vi "LabJackT4_Main.vi"() -> ()   [LabVIEW 2019]
uses:
  sub/enum_dev_id.ctl
  <vilib>/Analysis/baseanly.llb/Mean (DBL).vi
  <vilib>/Analysis/NI_AALBase.lvlib
panel:
  in  "logging_on":bool=TRUE
  out "status":bool
  out "TC_avg_degF":dbl format="%.1f"
  out "TC_avg_degC":dbl format="%.1f"
  out "array_ref_temp":dbl[](array[numeric]) caption="CJC" format="%_4g"
  out "Pressure":dbl
  in  "Tab Control":T1(tab)
  out "chart_pres":waveform(dbl)[](graph)=[{"t0"=timestamp(3772890114.31303 s since 1904-01-01), "dt"=1.0, "Y"=[0.8687935985565186]}, {"t0"=timestamp(3772890114.31303 s since 1904-01-01), "dt"=1.0, "Y"=[86.87935985565186]}, {"t0"=timestamp(3772890114.31303 s since 1904-01-01), "dt"=1.0, "Y"=[30.48853325313992]}, {"t0"=timestamp(3772890114.31303 s since 1904-01-01), "dt"=1.0, "Y"=[303.6385332531399]}]
  in  "SPTD25":string="AIN0"
  out "Chart degF":waveform(dbl)[](graph)
  out "Chart degC":waveform(dbl)[](graph)
  in  "LM34CAZ":string="AIN2"
  out "chart_ref_temp":waveform(dbl)[](graph)=[{"t0"=timestamp(3772890114.31303 s since 1904-01-01), "dt"=1.0, "Y"=[0.8687935985565186]}, {"t0"=timestamp(3772890114.31303 s since 1904-01-01), "dt"=1.0, "Y"=[86.87935985565186]}, {"t0"=timestamp(3772890114.31303 s since 1904-01-01), "dt"=1.0, "Y"=[30.48853325313992]}, {"t0"=timestamp(3772890114.31303 s since 1904-01-01), "dt"=1.0, "Y"=[303.6385332531399]}]
  out "chart_raw_v":waveform(dbl)[](graph)
  out "avg_data":dbl[](array[numeric])
  out "array_TC_degF":dbl[](array[numeric]) caption="TC degF" format="%_4g"
  out "array_TC_mV":dbl[](array[numeric]) caption="TC mV" format="%_4f"
  in  "amp_gain":dbl[](array[numeric])=[260.2, 260.0, 259.9, 259.8] format="%_4f"
  in  "amp_offset":dbl[](array[numeric])=[1.2648, 1.2687, 1.2357, 1.2546] format="%_5g"
  out "array_TC_degC":dbl[](array[numeric]) caption="TC degC" format="%_4g"
  in  "clear_chart":bool caption="Clear charts to start"
  in  "dev_id":T2=enum."192.168.24.185"
  out "SN":i32
  in  "conn_type":T3(ring)=enum."LJM_ctETHERNET"
  out "Last Meas. Time":timestamp format="%<%Y-%m-%d %H:%M:%S>T"
  in  "Read Rate (Hz)":dbl=0.1 format="%#_15g"
  out "iter":i32 caption="Meas. count"
  in  "Scan Rate (Hz)":dbl=5000.0 format="%#.3f"
  in  "stop":bool
  out "Error Message":string
  # "Pressure & Temperature of Outside gHe Tank"
  # "LabJack T4"
  # "psi"
  # "CH4"
  # "V"
  # "Bottom"
  # "degF"
  # "CH5"
  # "Right"
  # "CH6"
  # "Top"
  # "degC"
  # "CH7"
  # "K"
  # "Left"
  # "Average"
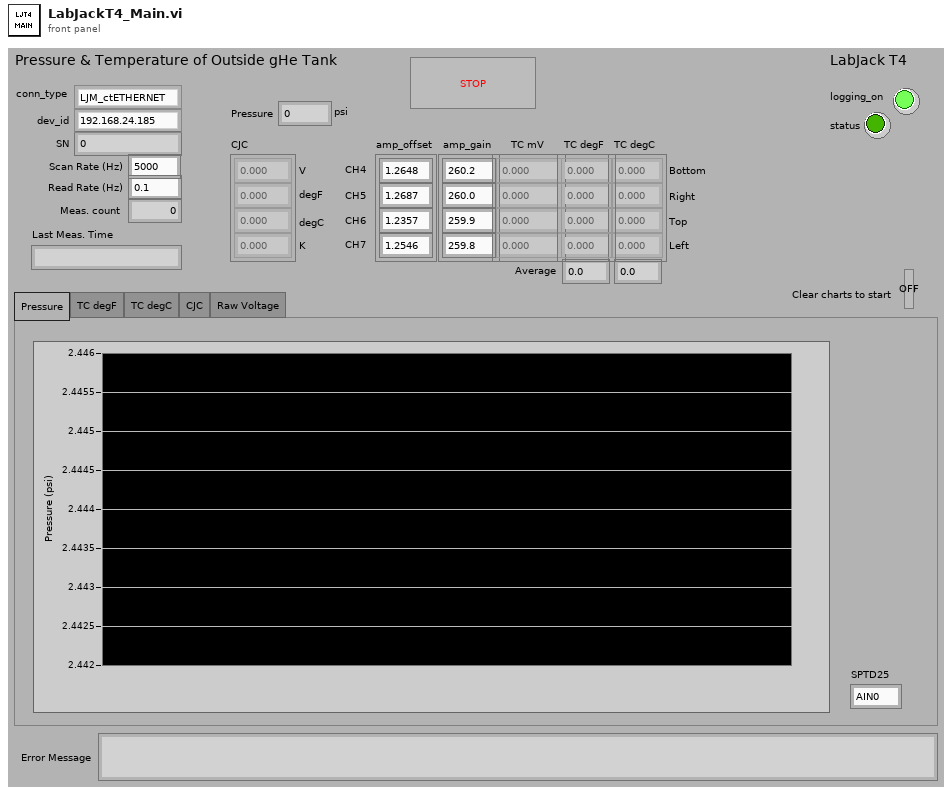
[diagram p1: front panel]
types:
  T1 = enum32{"Pressure", "TC degF", "TC degC", "CJC", "Raw Voltage"}
  T2 = typedef "enum_dev_id.ctl" = enum16{"LJM_idANY", "192.168.24.185", "10.0.0.176", "440017305"}
  T3 = enum16{"LJM_ctANY", "LJM_ctUSB", "LJM_ctETHERNET"}
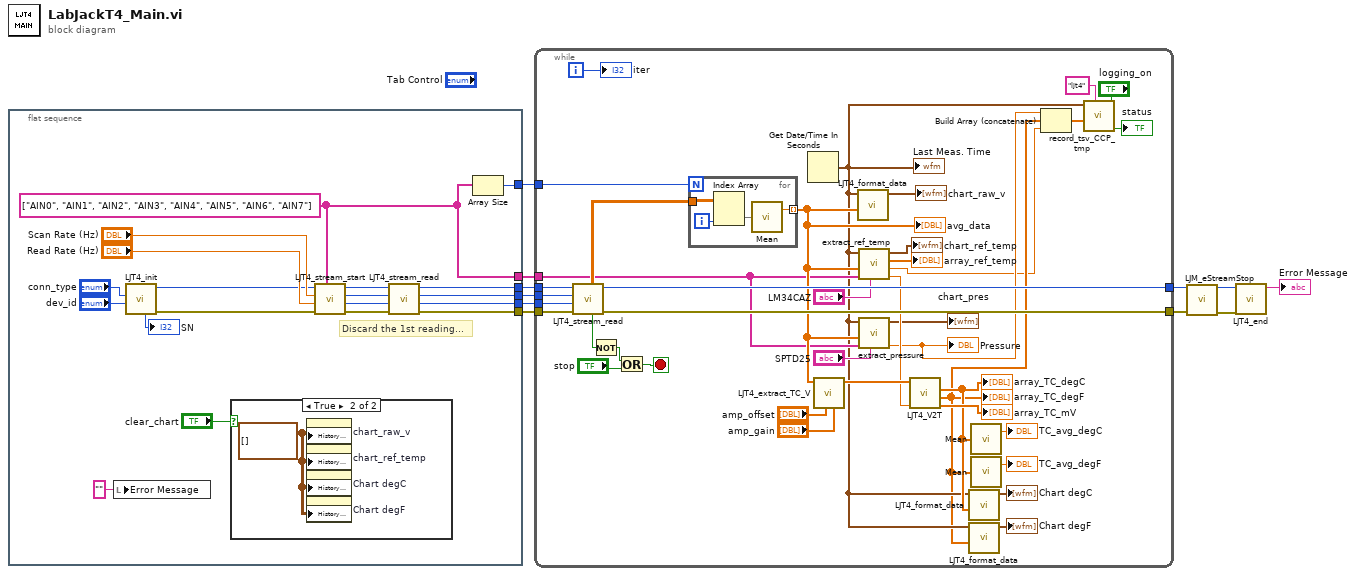
[diagram p0: block diagram]
diagram:
  n1 = flat-sequence {
    tunnel: [w18] -> w11
    tunnel: [w17] -> w10
    tunnel: [w14] -> w4
    tunnel: [w15] -> w3
    tunnel: [w23] -> w2
    tunnel: [w12] -> w1
    frame #0 {
      w12 = string[] ["AIN0", "AIN1", "AIN2", "AIN3", "AIN4", "AIN5", "AIN6", "AIN7"] ("Scan List")
      # "Discard the 1st reading..."
      n2 = local write "Error Message"("" ("Error Message")) -> ()
      n3 = call "LJT4_init.vi"("dev_id"="dev_id", "conn_type"="conn_type") -> ("error out"=w26:errorcluster, "Handle Out"=w24:i32, "SN"=→"SN":i32)  [unwired: 5 in, 2 out]
      n4 = case shown="True" "clear_chart" {
        frame False {
        }
        frame True {
          w29 = waveform(dbl)[][] [] ("History Data")
          n5 = property on="chart_raw_v" class="WFChart (strict)"("History Data"=w29) -> ()  [unwired: 2 in, 2 out]
          n6 = property on="chart_ref_temp" class="WFChart (strict)"("History Data"=w29) -> ()  [unwired: 2 in, 2 out]
          n7 = property on="Chart degC" class="WFChart (strict)"("History Data"=w29) -> ()  [unwired: 2 in, 2 out]
          n8 = property on="Chart degF" class="WFChart (strict)"("History Data"=w29) -> ()  [unwired: 2 in, 2 out]
        }
      }
      n9 = call "LJT4_stream_start.vi"("Scan List"=w12, "error in"=w26, "Read Rate (Hz)"="Read Rate (Hz)", "Scan Rate (Hz)"="Scan Rate (Hz)", "Handle in"=w24) -> ("error out"=w28:errorcluster, "NumReadAddresses"=w14:i32, "ScansPerRead Out"=w15:i32, "Handle out"=w16:i32)  [unwired: 1 in, 2 out]
      n10 = call "LJT4_stream_read.vi"("error in"=w28, "NumReadAddresses"=w14, "ScansPerRead"=w15, "Handle in"=w16) -> ("error out"=w18:errorcluster, "Handle Out"=w17:i32)  [unwired: 4 in, 2 out]
      n11 = Array Size(array=w12) -> (size(s)=w23:i32)
    }
  }
  n12 = while {
    tunnel: [w63] -> w8
    tunnel: w10 -> [w64]
    tunnel: w4 -> [w61]
    tunnel: w3 -> [w60]
    tunnel: w11 -> [w65]
    tunnel: [w62] -> w9
    tunnel: w2 -> [w57]
    tunnel: w1 -> [w43]
    i -> [w66]
    stop <- w67 stop-if-true
    n13 = call "LJT4_stream_read.vi"("error in"=w65, "NumReadAddresses"=w61, "ScansPerRead"=w60, "Handle in"=w64) -> ("error out"=w62:errorcluster, "Handle Out"=w63:i32, "status"=w59:bool, "data_out"=w58:dbl[][])  [unwired: 4 in]
    n14 = Not(x=w59) -> (.not. x?=w55:bool)
    n15 = Or(x=w55, y="stop") -> (x .or. y?=w67:bool)
    n16 = for {
      N: w57 -> [_]
      tunnel: w58 -> [w72]
      tunnel: [w69] -> w44 mode=indexing
      i -> [w71]
      n17 = Index Array(array=w72, index (col)=w71) -> (element=w70:dbl[])  [unwired: 1 in]
      n18 = call-poly <vilib>:"Mean.vi"("X"=w70) -> ("mean"=w69:dbl)  [unwired: 1 out]
    }
    "avg_data" <- w44
    n19 = Get Date/Time In Seconds() -> (seconds since 1Jan1904=w36:timestamp)
    "Last Meas. Time" <- w36
    n20 = call "LJT4_extract_TC_V.vi"("amp_gain"="amp_gain", "amp_offset"="amp_offset", "voltage_raw"=w44) -> ("voltage_TC"=w51:dbl[])  [unwired: 7 in, 1 out]
    n21 = call "LJT4_format_data.vi"("value_array"=w44, "time"=w36) -> ("waveform_array_A"=→"chart_raw_v":waveform(dbl)[])  [unwired: 9 in]
    n22 = call "extract_ref_temp.vi"("name"="LM34CAZ", "name_array"=w43, "value_array"=w44, "time"=w36) -> ("temp_K"=w50:dbl, "temp_F"=w30:dbl, "temp_array"=→"array_ref_temp":dbl[], "waveform_array"=→"chart_ref_temp":waveform(dbl)[])  [unwired: 4 in]
    n23 = call "extract_pressure.vi"("name"="SPTD25", "name_array"=w43, "value_array"=w44, "time"=w36) -> ("P"=w32:dbl, "waveform_array"=→"chart_pres":waveform(dbl)[])  [unwired: 4 in, 2 out]
    "Pressure" <- w32
    n24 = call "LJT4_V2T.vi"("CJC (K)"=w50, "voltage_array"=w51) -> ("array_mV"=→"array_TC_mV":dbl[], "array_T_F"=w31:dbl[], "array_T_C"=w40:dbl[])  [unwired: 6 in, 1 out]
    "array_TC_degC" <- w40
    "array_TC_degF" <- w31
    n25 = call "LJT4_format_data.vi"("value_array"=w40, "time"=w36) -> ("waveform_array_A"=→"Chart degC":waveform(dbl)[])  [unwired: 9 in]
    n26 = call "LJT4_format_data.vi"("value_array"=w31, "time"=w36) -> ("waveform_array_A"=→"Chart degF":waveform(dbl)[])  [unwired: 9 in]
    n27 = call-poly <vilib>:"Mean.vi"("X"=w40) -> ("mean"=→"TC_avg_degC":dbl)  [unwired: 1 out]
    n28 = call-poly <vilib>:"Mean.vi"("X"=w31) -> ("mean"=→"TC_avg_degF":dbl)  [unwired: 1 out]
    n29 = Build Array (concatenate)(w32, w31, w30) -> (w33:dbl[])
    n30 = call "record_tsv_CCP_tmp.vi"("logging_on"="logging_on", "folder_name"="ljt4", "value_array"=w33, "time"=w36) -> ("status"=→"status":bool)  [unwired: 6 in, 1 out]
    "iter" <- w66
  }
  n31 = call "LJM_eStreamStop.vi"("Handle In"=w8, "error in"=w9) -> ("Handle Out"=w6:i32, "error out"=w7:errorcluster)  [unwired: 12 in]
  n32 = call "LJT4_end.vi"("error in (no error)"=w7, "Handle Out"=w6) -> ("String"=→"Error Message":string)  [unwired: 9 in]
